vi "test-swerve-drive-kinematics-01.vi"() -> (3 "Test Passed":bool)   [LabVIEW 2019]
uses:
  <vilib>/Rock Robotics/WPI/ThirdParty/JAS_Junk/TrajLib/TypeDef/SWERVE_DRIVE_MODULE_STATE.ctl
  <vilib>/Rock Robotics/WPI/ThirdParty/JAS_Junk/TrajLib/TypeDef/ROTATION2D.ctl
  <vilib>/Rock Robotics/WPI/ThirdParty/JAS_Junk/TrajLib/Trajectory_Library.lvlib
panel:
  out "ModuleStates":T1[](array[typedef]) {"Angle"."SIN" format="%13.4f"; "Angle"."COS" format="%13.4f"; "Angle"."VALUE" format="%13.4f"}
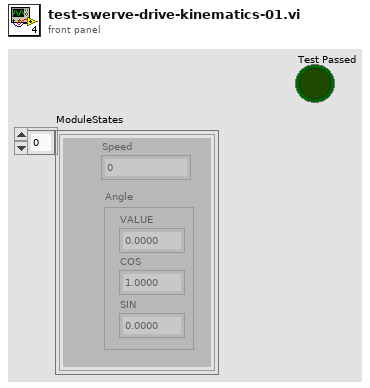
[diagram p1: front panel]
types:
  T1 = typedef "Trajectory_Library.lvlib/SWERVE_DRIVE_MODULE_STATE.ctl" = cluster{"Speed":dbl, "Angle":T2}
  T2 = typedef "Trajectory_Library.lvlib/ROTATION2D.ctl" = cluster{"VALUE":dbl, "COS":dbl, "SIN":dbl}
  T3 = typedef "Trajectory_Library.lvlib/TRANSLATION2D.ctl" = cluster{"X":dbl, "Y":dbl}
  T4 = typedef "Trajectory_Library.lvlib/SWERVE_DRIVE_KINEMATICS.ctl" = cluster{"NumModules":i32, "InverseKinematics":T5, "ForwardKinematics":T5, "Modules":T3[], "PrevCoR":T3, "SavedModuleStates":T1[]}
  T5 = typedef "NI_Matrix.lvlib/RealMatrix.ctl" = dbl[][]
  T6 = typedef "Trajectory_Library.lvlib/CHASSIS_SPEEDS.ctl" = cluster{"vX":dbl, "vY":dbl, "vOmega":dbl}
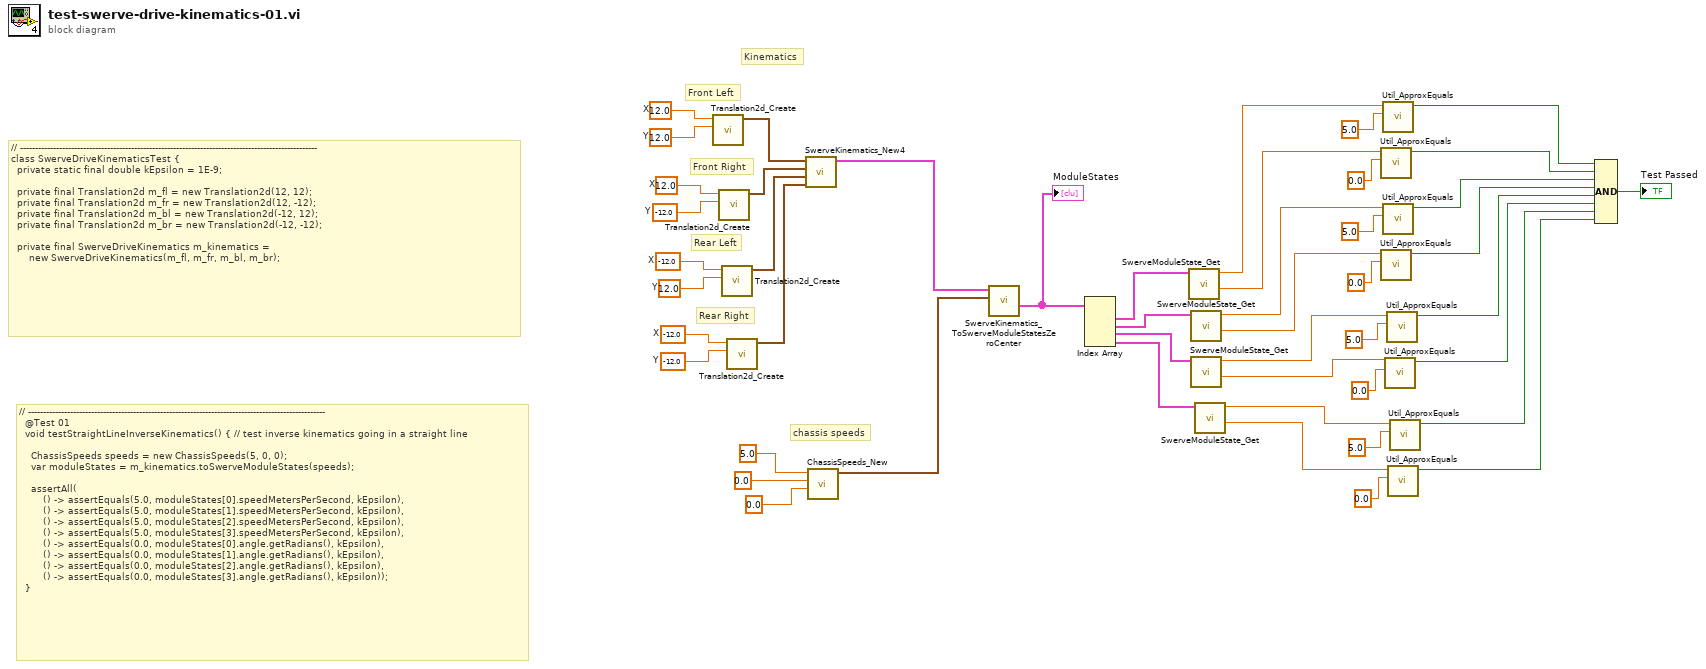
[diagram p0: block diagram]
diagram:
  w40 = -12.0  # X
  w39 = -12.0  # Y
  w38 = -12.0  # X
  w37 = 12.0  # Y
  w36 = 12.0  # X
  w35 = -12.0  # Y
  w34 = 12.0  # X
  w33 = 12.0  # Y
  # "// ---------------------------------------------------------------------------------------------------\n  @Test 01\n  void testStraightLineInverseKinematics() { // test inverse kinematics going in a straight line\n\n    ChassisSpeeds speeds = new ChassisSpeeds(5, 0, 0);\n    var moduleStates = m_kinematics.toSwerveModuleStates(speeds);\n\n    assertAll(\n        () -> assertEquals(5.0, moduleStates[0].speedMetersPerSecond, kEpsilon),\n        () -> assertEquals(5.0, moduleStates[1].speedMetersPerSecond, kEpsilon),\n        () -> assertEquals(5.0, moduleStates[2].speedMetersPerSecond, kEpsilon),\n        () -> assertEquals(5.0, moduleStates[3].speedMetersPerSecond, kEpsilon),\n        () -> assertEquals(0.0, moduleStates[0].angle.getRadians(), kEpsilon),\n        () -> assertEquals(0.0, moduleStates[1].angle.getRadians(), kEpsilon),\n        () -> assertEquals(0.0, moduleStates[2].angle.getRadians(), kEpsilon),\n        () -> assertEquals(0.0, moduleStates[3].angle.getRadians(), kEpsilon));\n  }"
  # "Kinematics"
  # "Rear Right"
  # "Rear Left"
  # "Front Right"
  # "Front Left"
  # "chassis speeds"
  # "// ---------------------------------------------------------------------------------------------------\nclass SwerveDriveKinematicsTest {\n  private static final double kEpsilon = 1E-9;\n\n  private final Translation2d m_fl = new Translation2d(12, 12);\n  private final Translation2d m_fr = new Translation2d(12, -12);\n  private final Translation2d m_bl = new Translation2d(-12, 12);\n  private final Translation2d m_br = new Translation2d(-12, -12);\n\n  private final SwerveDriveKinematics m_kinematics =\n      new SwerveDriveKinematics(m_fl, m_fr, m_bl, m_br);"
  n1 = call <vilib>:"Translation2d_Create.vi"("Y"=w33, "X"=w34) -> ("TRANSLATION"=w41:T3)  [unwired: 9 in]
  n2 = call <vilib>:"Translation2d_Create.vi"("Y"=w35, "X"=w36) -> ("TRANSLATION"=w42:T3)  [unwired: 9 in]
  n3 = call <vilib>:"Translation2d_Create.vi"("Y"=w37, "X"=w38) -> ("TRANSLATION"=w43:T3)  [unwired: 9 in]
  n4 = call <vilib>:"Translation2d_Create.vi"("Y"=w39, "X"=w40) -> ("TRANSLATION"=w44:T3)  [unwired: 9 in]
  n5 = call <vilib>:"SwerveKinematics_New4.vi"("wheel 3"=w44, "wheel 2"=w43, "wheel 1"=w42, "wheel 0"=w41) -> ("SWERVE_DRIVE_KINEMATICS"=w32:T4)  [unwired: 7 in]
  n6 = call <vilib>:"ChassisSpeeds_New.vi"("vAngular"=0.0, "vY"=0.0, "vX"=5.0) -> ("CHASSIS"=w31:T6)  [unwired: 8 in]
  n7 = call <vilib>:"SwerveKinematics_ToSwerveModuleStatesZeroCenter.vi"("ChassisSpeeds"=w31, "in SWERVE_DRIVE_KINEMATICS"=w32) -> ("ModuleStates"=w30:T1[])  [unwired: 8 in, 1 out]
  "ModuleStates" <- w30
  n8 = Index Array(array=w30) -> (element #1=w29:T1, element #2=w28:T1, element #3=w27:T1, element #4=w26:T1)  [unwired: 4 in]
  n9 = call <vilib>:"SwerveModuleState_Get.vi"("Desired State"=w29) -> ("Angle RADIANS"=w16:dbl, "Speed M/S"=w17:dbl)  [unwired: 9 in]
  n10 = call <vilib>:"SwerveModuleState_Get.vi"("Desired State"=w28) -> ("Angle RADIANS"=w14:dbl, "Speed M/S"=w15:dbl)  [unwired: 9 in]
  n11 = call <vilib>:"SwerveModuleState_Get.vi"("Desired State"=w27) -> ("Angle RADIANS"=w12:dbl, "Speed M/S"=w13:dbl)  [unwired: 9 in]
  n12 = call <vilib>:"SwerveModuleState_Get.vi"("Desired State"=w26) -> ("Angle RADIANS"=w10:dbl, "Speed M/S"=w11:dbl)  [unwired: 9 in]
  n13 = call <vilib>:"Util_ApproxEquals.vi"("Value 2"=0.0, "Value 1"=w16) -> ("ApproxEquals"=w8:bool)  [unwired: 9 in]
  n14 = call <vilib>:"Util_ApproxEquals.vi"("Value 2"=0.0, "Value 1"=w14) -> ("ApproxEquals"=w6:bool)  [unwired: 9 in]
  n15 = call <vilib>:"Util_ApproxEquals.vi"("Value 2"=5.0, "Value 1"=w17) -> ("ApproxEquals"=w9:bool)  [unwired: 9 in]
  n16 = call <vilib>:"Util_ApproxEquals.vi"("Value 2"=5.0, "Value 1"=w15) -> ("ApproxEquals"=w7:bool)  [unwired: 9 in]
  n17 = call <vilib>:"Util_ApproxEquals.vi"("Value 2"=0.0, "Value 1"=w12) -> ("ApproxEquals"=w4:bool)  [unwired: 9 in]
  n18 = call <vilib>:"Util_ApproxEquals.vi"("Value 2"=5.0, "Value 1"=w13) -> ("ApproxEquals"=w5:bool)  [unwired: 9 in]
  n19 = call <vilib>:"Util_ApproxEquals.vi"("Value 2"=0.0, "Value 1"=w10) -> ("ApproxEquals"=w2:bool)  [unwired: 9 in]
  n20 = call <vilib>:"Util_ApproxEquals.vi"("Value 2"=5.0, "Value 1"=w11) -> ("ApproxEquals"=w3:bool)  [unwired: 9 in]
  n21 = Compound Arithmetic op=AND(w9, w8, w7, w6, w5, w4, w3, w2) -> (→"Test Passed":bool)
